vi "Callback Change Direction.vi"(6 "Variant":variant, 8 "error in (no error)":errorcluster, 9 "old values":string[][](array[string]), 10 "object ref in":T2, 11 "Cluster":T3) -> (0 "error out":errorcluster)   [LabVIEW 2013, in "tag bus configurable plugin editor node.lvclass"]
uses:
  tag bus configurable plugin editor node.lvclass
  Table Manager/Cell Change.ctl
  Table Manager/object ref.ctl
  Configuration Editor/Classes/Engine Parent/Engine Parent Editor Node.lvclass
  Configuration Editor/Classes/Module editor node/module editor node.lvclass
  Permissions Enum.ctl
  module/configuration/tag bus configurable plugin module configuration.lvclass
  module/configuration/tag bus configurable plugin module configuration.lvclass/tag bus configurable plugin module configuration.ctl
  <vilib>/NI/Tag Bus Module Framework/channel/TBM channel.lvclass/TBM channel.ctl
  Table Manager.lvlib
  <vilib>/NI/Tag Bus Module Framework/channel/TBM channel.lvclass
  Table Manager/Table Manager.lvclass
panel:
  in  "Permissions":T1
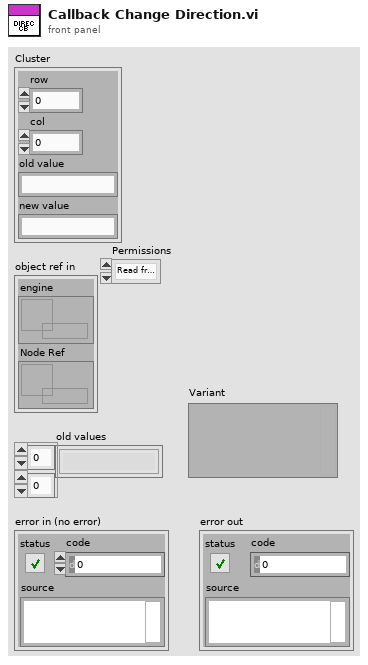
[diagram p1: front panel]
types:
  T1 = typedef "tag bus configurable plugin editor node.lvclass/Permissions Enum.ctl" = enum16{"Read from HW", "Write to HW"}
  T2 = typedef "Table Manager.lvlib/Table Manager.lvclass/object ref.ctl" = cluster{"engine":refnum<data-value>, "Node Ref":refnum<data-value>}
  T3 = typedef "Table Manager.lvlib/Cell Change.ctl" = cluster{"row":i32, "col":i32, "old value":string, "new value":string}
  T4 = typedef "TBM channel.lvclass/channel classification.ctl" = enum16{"input data", "output data", "processing parameter", "processing result"}
  T5 = typedef "tag bus configurable plugin module configuration.lvclass/Line.ctl" = cluster{"channel":refnum<class "TBM channel.lvclass">}
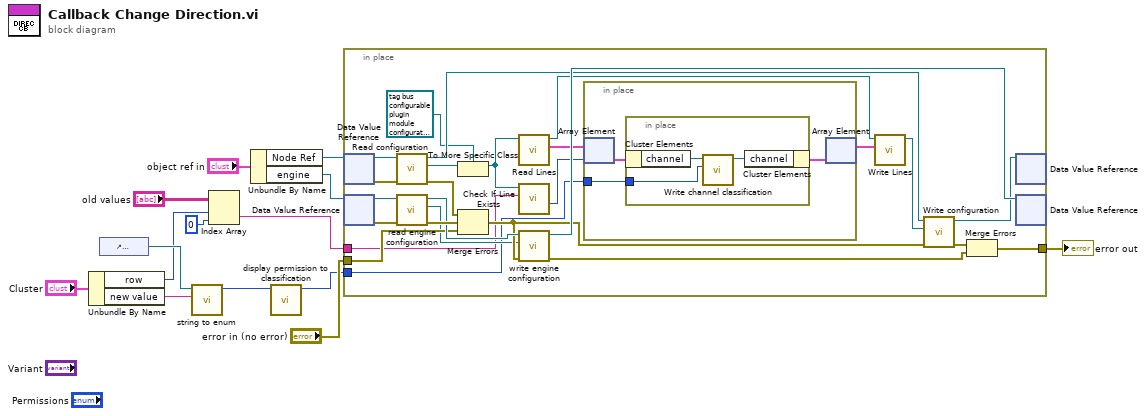
[diagram p0: block diagram]
diagram:
  n1 = Unbundle By Name("Cluster") -> ("row"=w1:i32, "new value"=w8:string)
  n2 = control-ref of="Permissions"() -> (w7:refnum<vi>)
  n3 = call "string to enum.vi"("String"=w8, "Enum"=w7) -> ("Value"=w6:i32)  [unwired: 8 in, 1 out]
  n4 = Index Array(array="old values", index (row)=w1, index (col)=0 ("disabled index (col)")) -> (element=w2:string)
  n5 = Unbundle By Name("object ref in") -> ("Node Ref"=w11:refnum<data-value>, "engine"=w10:refnum<data-value>)
  n6 = call "display permission to classification.vi"("display permissions"=w6) -> ("channel classification"=w5:T4)  [unwired: 10 in]
  n7 = in-place {
    in-place-border: [w32] -> w14
    in-place-border: "error in (no error)" -> [w25]
    in-place-border: w5 -> [w16]
    in-place-border: w2 -> [w15]
    n8 = in-place-dvr #1(w11) -> (w29:refnum<class "module editor node.lvclass">, w31:errorcluster)
    n9 = in-place-dvr #2(w10) -> (w39:refnum<class "Engine Parent Editor Node.lvclass">, w40:errorcluster)
    n10 = call-dynamic "Read configuration.vi"("error in"=w31, "NISE_CEF_serializable node in"=w29) -> ("error out"=w30:errorcluster, "configuration"=w27:refnum<class "NISE_CEF_serializable configuration.lvclass">, "NISE_CEF_serializable node out"=w28:refnum<class "module editor node.lvclass">)  [unwired: 7 in]
    n11 = call "read engine configuration.vi"("error in"=w40, "Engine Parent Editor Node in"=w39) -> ("error out"=w36:errorcluster, "engine configuration"=w24:refnum<class "engine configuration.lvclass">, "Engine Parent Editor Node out"=w35:refnum<class "Engine Parent Editor Node.lvclass">)  [unwired: 7 in]
    n12 = To More Specific Class(target class=refnum<class "tag bus configurable plugin module configuration.lvclass"> refnum ("tag bus configurable plugin module configuration"), reference=w27) -> (specific class reference=w20:refnum<class "tag bus configurable plugin module configuration.lvclass">)  [unwired: 1 in, 1 out]
    n13 = Merge Errors(w30, w36, w25) -> (w26:errorcluster)
    n14 = call "Read Lines.vi"("tag bus configurable plugin module configuration in"=w20) -> ("Lines"=w19:T5[], "tag bus configurable plugin module configuration out"=w21:refnum<class "tag bus configurable plugin module configuration.lvclass">)  [unwired: 8 in, 1 out]
    n15 = call-dynamic "Check If Line Exists.vi"("name to locate"=w15, "tag bus configurable plugin module configuration in"=w20) -> ("index"=w17:i32)  [unwired: 5 in, 4 out]
    n16 = call "write engine configuration.vi"("error in"=w26, "engine configuration"=w24, "Engine Parent Editor Node in"=w35) -> ("error out"=w34:errorcluster, "Engine Parent Editor Node out"=w38:refnum<class "Engine Parent Editor Node.lvclass">)  [unwired: 7 in]
    n17 = in-place {
      in-place-border: w16 -> [w41]
      n18 = in-place-array #3(w19, w17) -> (w43:T5)
      n19 = in-place {
        in-place-border: w41 -> [w44]
        n20 = in-place-cluster #4(w43) -> ("channel"=w46:refnum<class "TBM channel.lvclass">)
        n21 = call <vilib>:"Write channel classification.vi"("channel classification"=w44, "channel in"=w46) -> ("channel out"=w45:refnum<class "TBM channel.lvclass">)  [unwired: 8 in, 1 out]
        n22 = in-place-cluster #4("channel"=w45) -> (w42:T5)
      }
      n23 = in-place-array #3(w42) -> (w18:T5[])  [unwired: 1 out]
    }
    n24 = call "Write Lines.vi"("Lines"=w18, "tag bus configurable plugin module configuration in"=w21) -> ("tag bus configurable plugin module configuration out"=w22:refnum<class "tag bus configurable plugin module configuration.lvclass">)  [unwired: 8 in, 1 out]
    n25 = call-dynamic "Write configuration.vi"("error in"=w26, "configuration"=w22, "NISE_CEF_serializable node in"=w28) -> ("error out"=w33:errorcluster, "NISE_CEF_serializable node out"=w37:refnum<class "module editor node.lvclass">)  [unwired: 7 in]
    n26 = Merge Errors(w33, w34) -> (w32:errorcluster)
    n27 = in-place-dvr #1(w37) -> ()  [unwired: 2 out]
    n28 = in-place-dvr #2(w38) -> ()  [unwired: 2 out]
  }
  "error out" <- w14
